vi "Autonomous Independent.vi"() -> ()   [LabVIEW 2011]
doc: "This VI is called when autonomous begins, and will automatically be terminated when autonomous ends. You can carry out timed or sensor driven robot movement independently without needing to return to the caller."
uses:
  Autonomous Mode Selector.ctl
  <vilib>/Rock Robotics/WPI/Solenoid/WPI_SolenoidValue.ctl
  Shared/Autonomous Recording TypeDef.ctl
  Robot Global Data.vi
  Shooter Global.vi
  <vilib>/Rock Robotics/WPI/Solenoid/WPI_SolenoidSetEnum.vi
  <vilib>/addons/control/pid/pid.llb/PID (DBL).vi
  <vilib>/addons/control/pid/NI_PID_pid.lvlib
panel:
  in  "PID gains":T1={"proportional gain (Kc)"=0.01, "integral time (Ti, min)"=0.1, "derivative time (Td, min)"=0.0}
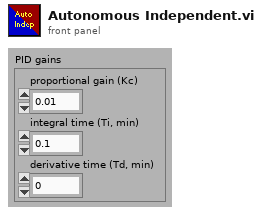
[diagram p1: front panel]
types:
  T1 = cluster{"proportional gain (Kc)":dbl, "integral time (Ti, min)":dbl, "derivative time (Td, min)":dbl}
  T2 = typedef "Autonomous Mode Selector.ctl" = enum16{"Shoot", "No Autonomous", "Shoot & Move"}
  T3 = typedef "WPI_DigitalInputDevRef.ctl" = cluster{"DevStatus":errorcluster, "DIO Channel":T4, "Digital Module":T5}
  T4 = typedef "FPGA_DIOChannel.ctl" = enum8{"DIO 1", "DIO 2", "DIO 3", "DIO 4", "DIO 5", "DIO 6", "DIO 7", "DIO 8", "DIO 9", "DIO 10", "DIO 11", "DIO 12", "DIO 13", "DIO 14", "Invalid"}
  T5 = typedef "FPGA_TypedefDigitalModule.ctl" = enum16{"Digital Module 1", "Digital Module 2"}
  T6 = enum16{"Off", "Open Loop Control", "Closed Loop Control", "Top Spin"}
  T7 = typedef "WPI_SolenoidValue.ctl" = enum16{"Off", "On", "Forward", "Reverse"}
  T8 = typedef "WPI_SolenoidDevRef.ctl" = cluster{"DevStatus":errorcluster, "Solenoid Module":T9, "Forward Solenoid Channel":T10, "Reverse Solenoid Channel":T10}
  T9 = typedef "FPGA_TypedefSolenoidModule.ctl" = enum16{"Solenoid Module 1", "Solenoid Module 2"}
  T10 = typedef "WPI_SolenoidChannel.ctl" = enum8{"Solenoid 1", "Solenoid 2", "Solenoid 3", "Solenoid 4", "Solenoid 5", "Solenoid 6", "Solenoid 7", "Solenoid 8", "Invalid"}
  T11 = typedef "WPI_RobotDriveDevRef.ctl" = cluster{"DevStatus":errorcluster, "Motors[]":T12[], "Square Inputs":bool, "Max Output":dbl, "Isochronous":bool}
  T12 = typedef "WPI_MotorControlDeviceRef.ctl" = cluster{"DeviceStatus":errorcluster, "Type":enum16{"PWM", "CAN"}, "PWM":cluster{"Digital Module":T5, "PWM Channel":T13, "DeadBand":T14}, "CAN":cluster{"Device Number":u8, "Control Mode":T15, "Semaphore":T16, "Max Vout":dbl}, "Invert":bool, "TransformRef":T17, "InvTransformRef":T17}
  T13 = typedef "FPGA_DIOPWMChannel.ctl" = enum8{"PWM 1", "PWM 2", "PWM 3", "PWM 4", "PWM 5", "PWM 6", "PWM 7", "PWM 8", "PWM 9", "PWM 10", "Invalid"}
  T14 = typedef "WPI_PWMDeadband.ctl" = cluster{"Name":string, "maxPositivePwm":i32, "minPositivePwm":i32, "centerPwm":i32, "maxNegativePwm":i32, "minNegativePwm":i32, "angularRange":u16}
  T15 = typedef "WPI_CANJaguar_ControlMode.ctl" = enum8{"Percent VBus", "Current", "Speed", "Position", "Voltage"}
  T16 = typedef "Semaphore RefNum" = refnum<k1>
  T17 = typedef "WPI_PWMTransform_ConPane.ctl" = refnum<vi>
  T18 = typedef "Autonomous Recording TypeDef.ctl" = cluster{"Left Drive Encoder":dbl, "Right Drive Encoder":dbl, "Shooter Mode":enum16{"Off", "Open Loop Control", "Closed Loop Control", "Top Spin"}, "Set RPM":dbl, "Set Motor Speed":dbl, "Horn":bool, "Shift Low":bool, "Shift High":bool, "Fire":bool, "Reset Encoders":bool}
  T19 = typedef "WPI_EncoderDevRef.ctl" = cluster{"DevStatus":errorcluster, "EncoderIndex":T20, "CounterIndex":T21, "DistancePerCount":dbl, "Decoding Type":T22}
  T20 = typedef "FPGA_EncoderIdx.ctl" = enum8{"Enc 0", "Enc 1", "Enc 2", "Enc 3", "Invalid"}
  T21 = typedef "FPGA_CounterCtrSystemIndex.ctl" = enum8{"Ctr 0", "Ctr 1", "Ctr 2", "Ctr 3", "Ctr 4", "Ctr 5", "Ctr 6", "Ctr 7", "Invalid"}
  T22 = typedef "WPI_EncoderType.ctl" = enum16{"1x", "2x", "4x"}
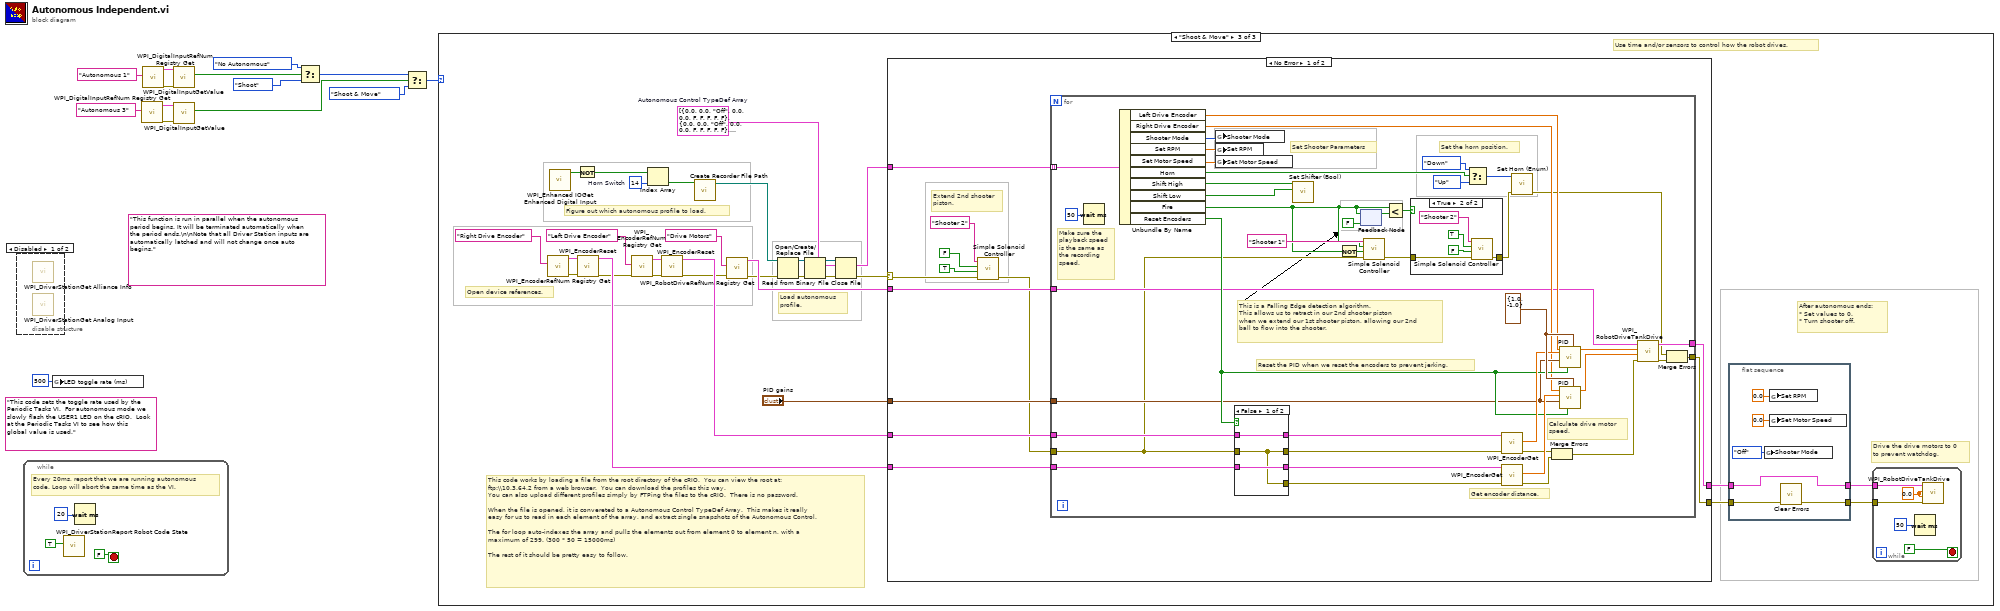
[diagram p0: block diagram]
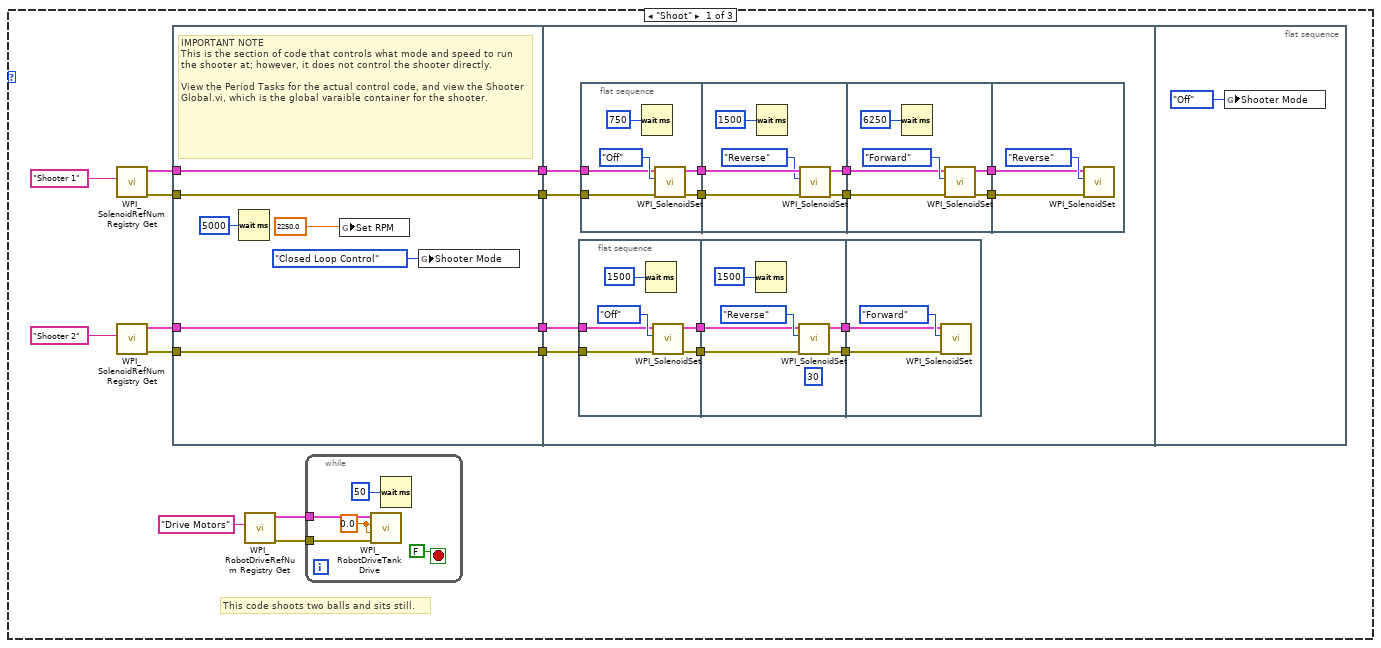
[diagram p3: hidden frame]
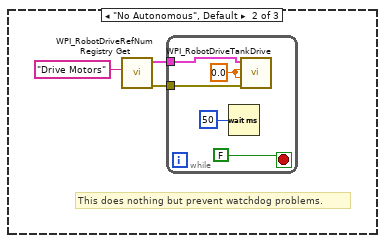
[diagram p4: hidden frame]
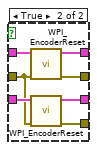
[diagram p6: hidden frame]
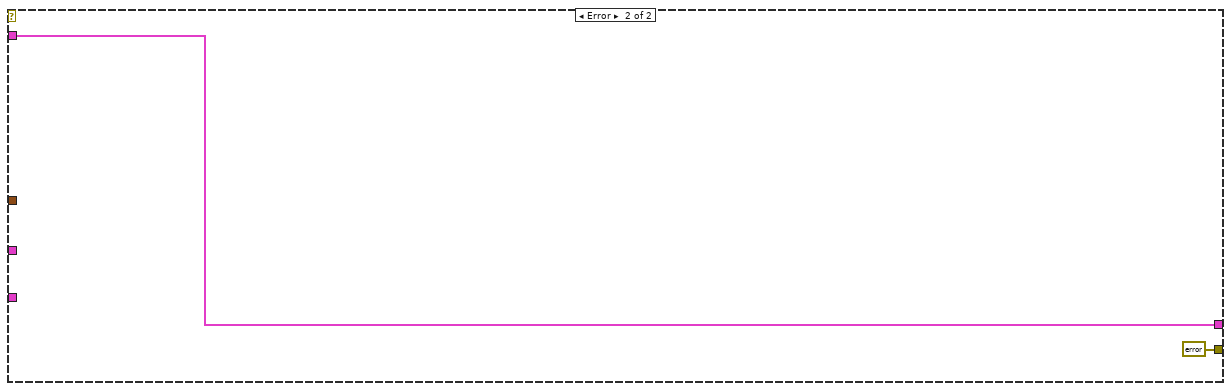
[diagram p7: hidden frame]
diagram:
  (unwired) "This code sets the toggle rate used by the Periodic Tasks VI.  For autonomous mode we slowly flash the USER1 LED on the cRIO.  Look at the Periodic Tasks VI to see how this global value is used."
  (unwired) "This function is run in parallel when the autonomous period begins. It will be terminated automatically when the period ends.\n\nNote that all Driver Station inputs are automatically latched and will not change once auto begins."
  # "Use time and/or sensors to control how the robot drives."
  n1 = disable-structure shown="Disabled" {
    frame Disabled {
      n2 = call <vilib>:"WPI_DriverStationGet Alliance Info.vi"() -> ()  [unwired: 12 out]
      n3 = call <vilib>:"WPI_DriverStationGet Analog Input.vi"() -> ()  [unwired: 12 out]
    }
    frame Enabled {
    }
  }
  n4 = while {
    stop <- FALSE stop-if-true
    # "Every 20ms, report that we are running autonomous\ncode. Loop will abort the same time as the VI."
    n5 = call <vilib>:"WPI_DriverStationReport Robot Code State.vi"("Autonomous"=TRUE) -> ()  [unwired: 10 in, 1 out]
    n6 = Wait (ms)(milliseconds to wait=u32 20) -> ()  [unwired: 1 out]
  }
  n7 = global write "Robot Global Data.vi" "LED toggle rate (ms)"(u32 500 ("LED ms toggle rate")) -> ()
  n8 = call <vilib>:"WPI_DigitalInputRefNum Registry Get.vi"("refnum name"="Autonomous 3") -> ("error out"=w9:errorcluster, "DigitalInputDevRef"=w8:T3)  [unwired: 9 in]
  n9 = call <vilib>:"WPI_DigitalInputRefNum Registry Get.vi"("refnum name"="Autonomous 1") -> ("error out"=w11:errorcluster, "DigitalInputDevRef"=w10:T3)  [unwired: 9 in]
  n10 = call <vilib>:"WPI_DigitalInputGetValue.vi"("error in (no error)"=w11, "DigitalInputDevRef"=w10) -> ("Value"=w7:bool)  [unwired: 7 in, 2 out]
  n11 = call <vilib>:"WPI_DigitalInputGetValue.vi"("error in (no error)"=w9, "DigitalInputDevRef"=w8) -> ("Value"=w2:bool)  [unwired: 7 in, 2 out]
  n12 = Select(t=Autonomous_Mode_Selector."No Autonomous", s=w7, f=Autonomous_Mode_Selector."Shoot") -> (s? t:f=w3:T2)
  n13 = Select(t=w3, s=w2, f=Autonomous_Mode_Selector."Shoot & Move") -> (s? t:f=w1:T2)
  n14 = case shown="\"Shoot & Move\"" w1 {
    frame "Shoot" {
      # "This code shoots two balls and sits still."
      n15 = call <vilib>:"WPI_SolenoidRefNum Registry Get.vi"("refnum name"="Shooter 1") -> ("error out"=w22:errorcluster, "SolenoidDevRef"=w24:T8)  [unwired: 9 in]
      n16 = call <vilib>:"WPI_SolenoidRefNum Registry Get.vi"("refnum name"="Shooter 2") -> ("error out"=w18:errorcluster, "SolenoidDevRef"=w20:T8)  [unwired: 9 in]
      n17 = flat-sequence {
        tunnel: [w34] -> w25
        tunnel: w24 -> [w34]
        tunnel: [w33] -> w23
        tunnel: w22 -> [w33]
        tunnel: [w32] -> w21
        tunnel: w20 -> [w32]
        tunnel: [w31] -> w19
        tunnel: w18 -> [w31]
        tunnel: w25 -> [w41]
        tunnel: w23 -> [w40]
        tunnel: w21 -> [w39]
        tunnel: w19 -> [w38]
        frame #0 {
          # "IMPORTANT NOTE\nThis is the section of code that controls what mode and speed to run the shooter at; however, it does not control the shooter directly.\n\nView the Period Tasks for the actual control code, and view the Shooter Global.vi, which is the global varaible container for the shooter."
          n18 = Wait (ms)(milliseconds to wait=u32 5000) -> ()  [unwired: 1 out]
          n19 = global write "Shooter Global.vi" "Set RPM"(2250.0 ("Output")) -> ()
          n20 = global write "Shooter Global.vi" "Shooter Mode"(T6."Closed Loop Control" ("Shooter Mode")) -> ()
        }
        frame #1 {
          n21 = flat-sequence {
            tunnel: w39 -> [w56]
            tunnel: w38 -> [w55]
            tunnel: [w53] -> w45
            tunnel: [w52] -> w44
            tunnel: w45 -> [w61]
            tunnel: w44 -> [w60]
            tunnel: [w59] -> w43
            tunnel: [w58] -> w42
            tunnel: w43 -> [w65]
            tunnel: w42 -> [w64]
            frame #0 {
              n22 = Wait (ms)(milliseconds to wait=u32 1500) -> ()  [unwired: 1 out]
              n23 = call-poly <vilib>:"WPI_SolenoidSet.vi"("error in (no error)"=w55, "Value"=WPI_SolenoidValue."Off", "SolenoidDevRef"=w56) -> ("error out"=w52:errorcluster, "SolenoidDevRef"=w53:T8)  [unwired: 7 in]
            }
            frame #1 {
              (unwired) 30 ("y")
              n24 = Wait (ms)(milliseconds to wait=u32 1500) -> ()  [unwired: 1 out]
              n25 = call-poly <vilib>:"WPI_SolenoidSet.vi"("error in (no error)"=w60, "Value"=WPI_SolenoidValue."Reverse", "SolenoidDevRef"=w61) -> ("error out"=w58:errorcluster, "SolenoidDevRef"=w59:T8)  [unwired: 7 in]
            }
            frame #2 {
              n26 = call-poly <vilib>:"WPI_SolenoidSet.vi"("error in (no error)"=w64, "Value"=WPI_SolenoidValue."Forward", "SolenoidDevRef"=w65) -> ()  [unwired: 7 in, 2 out]
            }
          }
          n27 = flat-sequence {
            tunnel: w41 -> [w71]
            tunnel: w40 -> [w70]
            tunnel: [w68] -> w51
            tunnel: [w67] -> w50
            tunnel: w51 -> [w78]
            tunnel: w50 -> [w77]
            tunnel: [w74] -> w49
            tunnel: [w73] -> w48
            tunnel: w49 -> [w83]
            tunnel: w48 -> [w82]
            tunnel: [w80] -> w47
            tunnel: [w79] -> w46
            tunnel: w47 -> [w86]
            tunnel: w46 -> [w85]
            frame #0 {
              n28 = Wait (ms)(milliseconds to wait=u32 750) -> ()  [unwired: 1 out]
              n29 = call-poly <vilib>:"WPI_SolenoidSet.vi"("error in (no error)"=w70, "Value"=WPI_SolenoidValue."Off", "SolenoidDevRef"=w71) -> ("error out"=w67:errorcluster, "SolenoidDevRef"=w68:T8)  [unwired: 7 in]
            }
            frame #1 {
              n30 = Wait (ms)(milliseconds to wait=u32 1500) -> ()  [unwired: 1 out]
              n31 = call-poly <vilib>:"WPI_SolenoidSet.vi"("error in (no error)"=w77, "Value"=WPI_SolenoidValue."Reverse", "SolenoidDevRef"=w78) -> ("error out"=w73:errorcluster, "SolenoidDevRef"=w74:T8)  [unwired: 7 in]
            }
            frame #2 {
              n32 = Wait (ms)(milliseconds to wait=u32 6250) -> ()  [unwired: 1 out]
              n33 = call-poly <vilib>:"WPI_SolenoidSet.vi"("error in (no error)"=w82, "Value"=WPI_SolenoidValue."Forward", "SolenoidDevRef"=w83) -> ("error out"=w79:errorcluster, "SolenoidDevRef"=w80:T8)  [unwired: 7 in]
            }
            frame #3 {
              n34 = call-poly <vilib>:"WPI_SolenoidSet.vi"("error in (no error)"=w85, "Value"=WPI_SolenoidValue."Reverse", "SolenoidDevRef"=w86) -> ()  [unwired: 7 in, 2 out]
            }
          }
        }
        frame #2 {
          n35 = global write "Shooter Global.vi" "Shooter Mode"(T6."Off" ("Shooter Mode")) -> ()
        }
      }
      n36 = call <vilib>:"WPI_RobotDriveRefNum Registry Get.vi"("refnum name"="Drive Motors") -> ("error out"=w29:errorcluster, "RobotDriveDevRef"=w28:T11)  [unwired: 9 in]
      n37 = while {
        tunnel: w29 -> [w91]
        tunnel: w28 -> [w90]
        stop <- FALSE stop-if-true
        w89 = 0.0 ("Left axis value")
        n38 = call <vilib>:"WPI_RobotDriveTankDrive.vi"("error in (no error)"=w91, "Right axis value"=w89, "Left axis value"=w89, "RobotDriveDevRef"=w90) -> ()  [unwired: 6 in, 2 out]
        n39 = Wait (ms)(milliseconds to wait=u32 50) -> ()  [unwired: 1 out]
      }
    }
    frame "No Autonomous", Default {
      # "This does nothing but prevent watchdog problems."
      n40 = call <vilib>:"WPI_RobotDriveRefNum Registry Get.vi"("refnum name"="Drive Motors") -> ("error out"=w94:errorcluster, "RobotDriveDevRef"=w95:T11)  [unwired: 9 in]
      n41 = while {
        tunnel: w95 -> [w101]
        tunnel: w94 -> [w97]
        stop <- FALSE stop-if-true
        w100 = 0.0 ("Left axis value")
        n42 = Wait (ms)(milliseconds to wait=u32 50) -> ()  [unwired: 1 out]
        n43 = call <vilib>:"WPI_RobotDriveTankDrive.vi"("error in (no error)"=w97, "Right axis value"=w100, "Left axis value"=w100, "RobotDriveDevRef"=w101) -> ()  [unwired: 6 in, 2 out]
      }
    }
    frame "Shoot & Move" {
      w108 = 14  # Horn Switch
      w115 = T18[] [{"Left Drive Encoder"=0.0, "Right Drive Encoder"=0.0, "Shooter Mode"=enum."Off", "Set RPM"=0.0, "Set Motor Speed"=0.0, "Horn"=FALSE, "Shift Low"=FALSE, "Shift High"=FALSE, "Fire"=FALSE, "Reset Encoders"=FALSE}, {"Left Drive Encoder"=0.0, "Right Drive Encoder"=0.0, "Shooter Mode"=enum."Off", "Set RPM"=0.0, "Set Motor Speed"=0.0, "Horn"=FALSE, "Shift Low"=FALSE, "Shift High"=FALSE, "Fire"=FALSE, "Reset Encoders"=FALSE}, {"Left Drive Encoder"=0.0, "Right Drive Encoder"=0.0, "Shooter Mode"=enum."Off", "Set RPM"=0.0, "Set Motor Speed"=0.0, "Horn"=FALSE, "Shift Low"=FALSE, "Shift High"=FALSE, "Fire"=FALSE, "Reset Encoders"=FALSE}, {"Left Drive Encoder"=0.0, "Right Drive Encoder"=0.0, "Shooter Mode"=enum."Off", "Set RPM"=0.0, "Set Motor Speed"=0.0, "Horn"=FALSE, "Shift Low"=FALSE, "Shift High"=FALSE, "Fire"=FALSE, "Reset Encoders"=FALSE}, {"Left Drive Encoder"=0.0, "Right Drive Encoder"=0.0, "Shooter Mode"=enum."Off", "Set RPM"=0.0, "Set Motor Speed"=0.0, "Horn"=FALSE, "Shift Low"=FALSE, "Shift High"=FALSE, "Fire"=FALSE, "Reset Encoders"=FALSE}, {"Left Drive Encoder"=0.0, "Right Drive Encoder"=0.0, "Shooter Mode"=enum."Off", "Set RPM"=0.0, "Set Motor Speed"=0.0, "Horn"=FALSE, "Shift Low"=FALSE, "Shift High"=FALSE, "Fire"=FALSE, "Reset Encoders"=FALSE}, {"Left Drive Encoder"=0.0, "Right Drive Encoder"=0.0, "Shooter Mode"=enum."Off", "Set RPM"=0.0, "Set Motor Speed"=0.0, "Horn"=FALSE, "Shift Low"=FALSE, "Shift High"=FALSE, "Fire"=FALSE, "Reset Encoders"=FALSE}, {"Left Drive Encoder"=0.0, "Right Drive Encoder"=0.0, "Shooter Mode"=enum."Off", "Set RPM"=0.0, "Set Motor Speed"=0.0, "Horn"=FALSE, "Shift Low"=FALSE, "Shift High"=FALSE, "Fire"=FALSE, "Reset Encoders"=FALSE}, {"Left Drive Encoder"=0.0, "Right Drive Encoder"=0.0, "Shooter Mode"=enum."Off", "Set RPM"=0.0, "Set Motor Speed"=0.0, "Horn"=FALSE, "Shift Low"=FALSE, "Shift High"=FALSE, "Fire"=FALSE, "Reset Encoders"=FALSE}, {"Left Drive Encoder"=0.0, "Right Drive Encoder"=0.0, "Shooter Mode"=enum."Off", "Set RPM"=0.0, "Set Motor Speed"=0.0, "Horn"=FALSE, "Shift Low"=FALSE, "Shift High"=FALSE, "Fire"=FALSE, "Reset Encoders"=FALSE}, {"Left Drive Encoder"=0.0, "Right Drive Encoder"=0.0, "Shooter Mode"=enum."Off", "Set RPM"=0.0, "Set Motor Speed"=0.0, "Horn"=FALSE, "Shift Low"=FALSE, "Shift High"=FALSE, "Fire"=FALSE, "Reset Encoders"=FALSE}, {"Left Drive Encoder"=0.0, "Right Drive Encoder"=0.0, "Shooter Mode"=enum."Off", "Set RPM"=0.0, "Set Motor Speed"=0.0, "Horn"=FALSE, "Shift Low"=FALSE, "Shift High"=FALSE, "Fire"=FALSE, "Reset Encoders"=FALSE}, {"Left Drive Encoder"=0.0, "Right Drive Encoder"=0.0, "Shooter Mode"=enum."Off", "Set RPM"=0.0, "Set Motor Speed"=0.0, "Horn"=FALSE, "Shift Low"=FALSE, "Shift High"=FALSE, "Fire"=FALSE, "Reset Encoders"=FALSE}, {"Left Drive Encoder"=0.0, "Right Drive Encoder"=0.0, "Shooter Mode"=enum."Off", "Set RPM"=0.0, "Set Motor Speed"=0.0, "Horn"=FALSE, "Shift Low"=FALSE, "Shift High"=FALSE, "Fire"=FALSE, "Reset Encoders"=FALSE}, {"Left Drive Encoder"=0.0, "Right Drive Encoder"=0.0, "Shooter Mode"=enum."Off", "Set RPM"=0.0, "Set Motor Speed"=0.0, "Horn"=FALSE, "Shift Low"=FALSE, "Shift High"=FALSE, "Fire"=FALSE, "Reset Encoders"=FALSE}, {"Left Drive Encoder"=0.0, "Right Drive Encoder"=0.0, "Shooter Mode"=enum."Off", "Set RPM"=0.0, "Set Motor Speed"=0.0, "Horn"=FALSE, "Shift Low"=FALSE, "Shift High"=FALSE, "Fire"=FALSE, "Reset Encoders"=FALSE}, {"Left Drive Encoder"=0.0, "Right Drive Encoder"=0.0, "Shooter Mode"=enum."Off", "Set RPM"=0.0, "Set Motor Speed"=0.0, "Horn"=FALSE, "Shift Low"=FALSE, "Shift High"=FALSE, "Fire"=FALSE, "Reset Encoders"=FALSE}, {"Left Drive Encoder"=0.0, "Right Drive Encoder"=0.0, "Shooter Mode"=enum."Off", "Set RPM"=0.0, "Set Motor Speed"=0.0, "Horn"=FALSE, "Shift Low"=FALSE, "Shift High"=FALSE, "Fire"=FALSE, "Reset Encoders"=FALSE}, {"Left Drive Encoder"=0.0, "Right Drive Encoder"=0.0, "Shooter Mode"=enum."Off", "Set RPM"=0.0, "Set Motor Speed"=0.0, "Horn"=FALSE, "Shift Low"=FALSE, "Shift High"=FALSE, "Fire"=FALSE, "Reset Encoders"=FALSE}, {"Left Drive Encoder"=0.0, "Right Drive Encoder"=0.0, "Shooter Mode"=enum."Off", "Set RPM"=0.0, "Set Motor Speed"=0.0, "Horn"=FALSE, "Shift Low"=FALSE, "Shift High"=FALSE, "Fire"=FALSE, "Reset Encoders"=FALSE}, {"Left Drive Encoder"=0.0, "Right Drive Encoder"=0.0, "Shooter Mode"=enum."Off", "Set RPM"=0.0, "Set Motor Speed"=0.0, "Horn"=FALSE, "Shift Low"=FALSE, "Shift High"=FALSE, "Fire"=FALSE, "Reset Encoders"=FALSE}, {"Left Drive Encoder"=0.0, "Right Drive Encoder"=0.0, "Shooter Mode"=enum."Off", "Set RPM"=0.0, "Set Motor Speed"=0.0, "Horn"=FALSE, "Shift Low"=FALSE, "Shift High"=FALSE, "Fire"=FALSE, "Reset Encoders"=FALSE}, {"Left Drive Encoder"=0.0, "Right Drive Encoder"=0.0, "Shooter Mode"=enum."Off", "Set RPM"=0.0, "Set Motor Speed"=0.0, "Horn"=FALSE, "Shift Low"=FALSE, "Shift High"=FALSE, "Fire"=FALSE, "Reset Encoders"=FALSE}, {"Left Drive Encoder"=0.0, "Right Drive Encoder"=0.0, "Shooter Mode"=enum."Off", "Set RPM"=0.0, "Set Motor Speed"=0.0, "Horn"=FALSE, "Shift Low"=FALSE, "Shift High"=FALSE, "Fire"=FALSE, "Reset Encoders"=FALSE}, {"Left Drive Encoder"=0.0, "Right Drive Encoder"=0.0, "Shooter Mode"=enum."Off", "Set RPM"=0.0, "Set Motor Speed"=0.0, "Horn"=FALSE, "Shift Low"=FALSE, "Shift High"=FALSE, "Fire"=FALSE, "Reset Encoders"=FALSE}, {"Left Drive Encoder"=0.0, "Right Drive Encoder"=0.0, "Shooter Mode"=enum."Off", "Set RPM"=0.0, "Set Motor Speed"=0.0, "Horn"=FALSE, "Shift Low"=FALSE, "Shift High"=FALSE, "Fire"=FALSE, "Reset Encoders"=FALSE}, {"Left Drive Encoder"=0.0, "Right Drive Encoder"=0.0, "Shooter Mode"=enum."Off", "Set RPM"=0.0, "Set Motor Speed"=0.0, "Horn"=FALSE, "Shift Low"=FALSE, "Shift High"=FALSE, "Fire"=FALSE, "Reset Encoders"=FALSE}, {"Left Drive Encoder"=0.0, "Right Drive Encoder"=0.0, "Shooter Mode"=enum."Off", "Set RPM"=0.0, "Set Motor Speed"=0.0, "Horn"=FALSE, "Shift Low"=FALSE, "Shift High"=FALSE, "Fire"=FALSE, "Reset Encoders"=FALSE}, {"Left Drive Encoder"=0.0, "Right Drive Encoder"=0.0, "Shooter Mode"=enum."Off", "Set RPM"=0.0, "Set Motor Speed"=0.0, "Horn"=FALSE, "Shift Low"=FALSE, "Shift High"=FALSE, "Fire"=FALSE, "Reset Encoders"=FALSE}, {"Left Drive Encoder"=0.0, "Right Drive Encoder"=0.0, "Shooter Mode"=enum."Off", "Set RPM"=0.0, "Set Motor Speed"=0.0, "Horn"=FALSE, "Shift Low"=FALSE, "Shift High"=FALSE, "Fire"=FALSE, "Reset Encoders"=FALSE}, {"Left Drive Encoder"=0.0, "Right Drive Encoder"=0.0, "Shooter Mode"=enum."Off", "Set RPM"=0.0, "Set Motor Speed"=0.0, "Horn"=FALSE, "Shift Low"=FALSE, "Shift High"=FALSE, "Fire"=FALSE, "Reset Encoders"=FALSE}, {"Left Drive Encoder"=0.0, "Right Drive Encoder"=0.0, "Shooter Mode"=enum."Off", "Set RPM"=0.0, "Set Motor Speed"=0.0, "Horn"=FALSE, "Shift Low"=FALSE, "Shift High"=FALSE, "Fire"=FALSE, "Reset Encoders"=FALSE}, {"Left Drive Encoder"=0.0, "Right Drive Encoder"=0.0, "Shooter Mode"=enum."Off", "Set RPM"=0.0, "Set Motor Speed"=0.0, "Horn"=FALSE, "Shift Low"=FALSE, "Shift High"=FALSE, "Fire"=FALSE, "Reset Encoders"=FALSE}, {"Left Drive Encoder"=0.0, "Right Drive Encoder"=0.0, "Shooter Mode"=enum."Off", "Set RPM"=0.0, "Set Motor Speed"=0.0, "Horn"=FALSE, "Shift Low"=FALSE, "Shift High"=FALSE, "Fire"=FALSE, "Reset Encoders"=FALSE}, {"Left Drive Encoder"=0.0, "Right Drive Encoder"=0.0, "Shooter Mode"=enum."Off", "Set RPM"=0.0, "Set Motor Speed"=0.0, "Horn"=FALSE, "Shift Low"=FALSE, "Shift High"=FALSE, "Fire"=FALSE, "Reset Encoders"=FALSE}, {"Left Drive Encoder"=-1.7999999999999998, "Right Drive Encoder"=-1.7999999999999998, "Shooter Mode"=enum."Off", "Set RPM"=0.0, "Set Motor Speed"=0.0, "Horn"=FALSE, "Shift Low"=FALSE, "Shift High"=FALSE, "Fire"=FALSE, "Reset Encoders"=FALSE}, {"Left Drive Encoder"=-8.64, "Right Drive Encoder"=-6.12, "Shooter Mode"=enum."Off", "Set RPM"=0.0, "Set Motor Speed"=0.0, "Horn"=FALSE, "Shift Low"=FALSE, "Shift High"=FALSE, "Fire"=FALSE, "Reset Encoders"=FALSE}, {"Left Drive Encoder"=-14.399999999999999, "Right Drive Encoder"=-13.68, "Shooter Mode"=enum."Off", "Set RPM"=0.0, "Set Motor Speed"=0.0, "Horn"=FALSE, "Shift Low"=FALSE, "Shift High"=FALSE, "Fire"=FALSE, "Reset Encoders"=FALSE}, {"Left Drive Encoder"=-24.119999999999997, "Right Drive Encoder"=-27.36, "Shooter Mode"=enum."Off", "Set RPM"=0.0, "Set Motor Speed"=0.0, "Horn"=FALSE, "Shift Low"=FALSE, "Shift High"=FALSE, "Fire"=FALSE, "Reset Encoders"=FALSE}, {"Left Drive Encoder"=-36.36, "Right Drive Encoder"=0.0, "Shooter Mode"=enum."Off", "Set RPM"=0.0, "Set Motor Speed"=0.0, "Horn"=FALSE, "Shift Low"=FALSE, "Shift High"=FALSE, "Fire"=FALSE, "Reset Encoders"=FALSE}]  # Autonomous Control TypeDef Array
      # "After autonomous ends:\n* Set values to 0.\n* Turn shooter off."
      # "This code works by loading a file from the root directory of the cRIO.  You can view the root at:\nftp:\\\\10.3.64.2 from a web browser.  You can download the profiles this way.\nYou can also upload different profiles simply by FTPing the files to the cRIO.  There is no password.\n\nWhen the file is opened, it is convereted to a Autonomous Control TypeDef Array.  This makes it really\neasy for us to read in each element of the array, and extract single snapshots of the Autonomous Control.\n\nThe for loop auto-indexes the array and pulls the elements out from element 0 to element n, with a \nmaximum of 299. (300 * 50 = 15000ms)\n\nThe rest of it should be pretty easy to follow."
      # "Drive the drive motors to 0\nto prevent watchdog."
      # "Figure out which autonomous profile to load."
      # "Load autonomous\nprofile."
      # "Open device references."
      n44 = call <vilib>:"WPI_EncoderRefNum Registry Get.vi"("refnum name"="Right Drive Encoder") -> ("error out"=w129:errorcluster, "EncoderDevRef"=w126:T19)  [unwired: 9 in]
      n45 = call <vilib>:"WPI_Enhanced IOGet Enhanced Digital Input.vi"() -> ("Digital Input [1-16]"=w106:bool[])  [unwired: 10 in, 1 out]
      n46 = Not(x=w106) -> (.not. x?=w107:bool[])
      n47 = call <vilib>:"WPI_EncoderReset.vi"("error in (no error)"=w129, "EncoderDevRef"=w126) -> ("error out"=w110:errorcluster, "EncoderDevRef"=w124:T19)  [unwired: 8 out]
      n48 = call <vilib>:"WPI_EncoderRefNum Registry Get.vi"("error in (no error)"=w110, "refnum name"="Left Drive Encoder") -> ("error out"=w128:errorcluster, "EncoderDevRef"=w127:T19)  [unwired: 8 in]
      n49 = Index Array(array=w107, index=w108) -> (element=w109:bool)
      n50 = call <vilib>:"WPI_EncoderReset.vi"("error in (no error)"=w128, "EncoderDevRef"=w127) -> ("error out"=w111:errorcluster, "EncoderDevRef"=w125:T19)  [unwired: 8 out]
      n51 = call "Create Recorder File Path.vi"("T: Move_Shoot\nF: Shoot_Move"=w109) -> ("Path"=w105:path)  [unwired: 10 in]
      n52 = call <vilib>:"WPI_RobotDriveRefNum Registry Get.vi"("error in (no error)"=w111, "refnum name"="Drive Motors") -> ("error out"=w121:errorcluster, "RobotDriveDevRef"=w122:T11)  [unwired: 8 in]
      n53 = Open/Create/Replace File(file path (use dialog)=w105, error in=w121) -> (refnum out=w116:refnum<file>, error out=w117:errorcluster)  [unwired: 4 in, 1 out]
      n54 = Read from Binary File(5:w115, 8:w117, 11:w116) -> (0:w112:errorcluster, 2:w114:T18[], 3:w113:refnum<file>)  [unwired: 3 in, 1 out]
      n55 = Close File(refnum=w113, error in=w112) -> (error out=w104:errorcluster)  [unwired: 1 out]
      n56 = case shown="No Error" w104 {
        selector: w104 -> [w134 _]
        tunnel: w125 -> [w143 _]
        tunnel: w124 -> [w142 _]
        tunnel: "PID gains" -> [w141 _]
        tunnel: w122 -> [w140 w204]
        tunnel: [w139 w204] -> w118
        tunnel: w114 -> [w138 _]
        tunnel: [w132 errorcluster {"status"=FALSE, "code"=0, "source"=""} ("error IO")] -> w102
        frame No Error {
          # "Extend 2nd shooter\npiston."
          n57 = call "Simple Solenoid Controller.vi"("error in (no error)"=w134, "Reverse"=TRUE, "Forward"=FALSE, "refnum name"="Shooter 2") -> ("error out"=w133:errorcluster)  [unwired: 6 in, 1 out]
          n58 = for {
            tunnel: w138 -> [w154] mode=indexing
            tunnel: w143 -> [w180]
            tunnel: w142 -> [w179]
            tunnel: w141 -> [w175]
            tunnel: w140 -> [w172]
            tunnel: [w155] -> w139
            tunnel: w133 -> [w151]
            tunnel: [w144] -> w132
            w185 = cluster{"output high":dbl, "output low":dbl} {"output high"=1.0, "output low"=-1.0} ("output range")
            # "Calculate drive motor\nspeed."
            # "Get encoder distance."
            # "Set the horn position."
            # "This is a Falling Edge detection algorithm.\nThis allows us to retract in our 2nd shooter piston\nwhen we extend our 1st shooter piston, allowing our 2nd\nball to flow into the shooter."
            # "Reset the PID when we reset the encoders to prevent jerking."
            # "Set Shooter Parameters"
            # "Make sure the\nplayback speed\nis the same as\nthe recording\nspeed."
            n59 = Wait (ms)(milliseconds to wait=u32 50) -> ()  [unwired: 1 out]
            n60 = Unbundle By Name(w154) -> ("Left Drive Encoder"=w174:dbl, "Right Drive Encoder"=w173:dbl, "Shooter Mode"=w156:T6, "Set RPM"=w158:dbl, "Set Motor Speed"=w157:dbl, "Horn"=w159:bool, "Shift High"=w171:bool, "Shift Low"=w170:bool, "Fire"=w165:bool, "Reset Encoders"=w176:bool)
            n61 = global write "Shooter Global.vi" "Shooter Mode"(w156) -> ()
            n62 = global write "Shooter Global.vi" "Set RPM"(w158) -> ()
            n63 = global write "Shooter Global.vi" "Set Motor Speed"(w157) -> ()
            n64 = case shown="False" w176 {
              tunnel: w180 -> [w195 w202]
              tunnel: w179 -> [w194 w201]
              tunnel: [w194 w200] -> w178
              tunnel: [w195 w199] -> w177
              tunnel: w151 -> [w193 w198]
              tunnel: [w193 w197] -> w153
              tunnel: [w193 w196] -> w152
              frame False {
              }
              frame True {
                n65 = call <vilib>:"WPI_EncoderReset.vi"("error in (no error)"=w198, "EncoderDevRef"=w202) -> ("error out"=w197:errorcluster, "EncoderDevRef"=w199:T19)  [unwired: 8 out]
                n66 = call <vilib>:"WPI_EncoderReset.vi"("error in (no error)"=w198, "EncoderDevRef"=w201) -> ("error out"=w196:errorcluster, "EncoderDevRef"=w200:T19)  [unwired: 8 out]
              }
            }
            n67 = call "Set Shifter (Bool).vi"("Low"=w170, "High"=w171) -> ()  [unwired: 9 in, 1 out]
            n68 = Not(x=w165) -> (.not. x?=w168:bool)
            n69 = feedback-in #1(w165) -> ()
            n70 = feedback #1(FALSE) -> (w164:bool)
            n71 = call "Simple Solenoid Controller.vi"("error in (no error)"=w151, "Reverse"=w168, "Forward"=w165, "refnum name"="Shooter 1") -> ("error out"=w167:errorcluster)  [unwired: 6 in, 1 out]
            n72 = Less?(x=w165, y=w164) -> (x < y?=w163:bool)
            n73 = case shown="True" w163 {
              tunnel: w167 -> [w187 w189]
              tunnel: [w187 w188] -> w146
              frame False {
              }
              frame True {
                n74 = call "Simple Solenoid Controller.vi"("error in (no error)"=w189, "Reverse"=FALSE, "Forward"=TRUE, "refnum name"="Shooter 2") -> ("error out"=w188:errorcluster)  [unwired: 6 in, 1 out]
              }
            }
            n75 = Select(t=enum16{"Down", "Up"}."Down" ("Horn"), s=w159, f=enum16{"Down", "Up"}."Up") -> (s? t:f=w162:enum16{"Down", "Up"})
            n76 = call <vilib>:"WPI_EncoderGet.vi"("error in (no error)"=w153, "EncoderDevRef"=w177) -> ("error out"=w150:errorcluster, "Distance"=w181:dbl)  [unwired: 8 out]
            n77 = call <vilib>:"WPI_EncoderGet.vi"("error in (no error)"=w152, "EncoderDevRef"=w178) -> ("error out"=w149:errorcluster, "Distance"=w182:dbl)  [unwired: 8 out]
            n78 = call "Set Horn (Enum).vi"("error in (no error)"=w146, "Horn"=w162) -> ("error out"=w145:errorcluster)  [unwired: 9 in]
            n79 = Merge Errors(w150, w149) -> (w148:errorcluster)
            n80 = call-poly <vilib>:"PID.vi"("reinitialize? (F)"=w176, "output range"=w185, "PID gains"=w175, "process variable"=w181, "setpoint"=w174) -> ("output"=w184:dbl)  [unwired: 5 in, 1 out]
            n81 = call-poly <vilib>:"PID.vi"("reinitialize? (F)"=w176, "output range"=w185, "PID gains"=w175, "process variable"=w182, "setpoint"=w173) -> ("output"=w183:dbl)  [unwired: 5 in, 1 out]
            n82 = call <vilib>:"WPI_RobotDriveTankDrive.vi"("error in (no error)"=w148, "Right axis value"=w183, "Left axis value"=w184, "RobotDriveDevRef"=w172) -> ("error out"=w147:errorcluster, "RobotDriveDevRef"=w155:T11)  [unwired: 6 in]
            n83 = Merge Errors(w145, w147) -> (w144:errorcluster)
          }
        }
        frame Error {
        }
      }
      n84 = flat-sequence {
        tunnel: [w208] -> w119
        tunnel: w118 -> [w208]
        tunnel: [w205] -> w103
        tunnel: w102 -> [w206]
        frame #0 {
          n85 = global write "Shooter Global.vi" "Shooter Mode"(T6."Off" ("Shooter Mode")) -> ()
          n86 = global write "Shooter Global.vi" "Set RPM"(0.0 ("Set RPM")) -> ()
          n87 = global write "Shooter Global.vi" "Set Motor Speed"(0.0 ("Set Motor Speed")) -> ()
          n88 = call <vilib>:"Clear Errors.vi"("error in (no error)"=w206) -> ("error out"=w205:errorcluster)  [unwired: 6 in]
        }
      }
      n89 = while {
        tunnel: w119 -> [w215]
        tunnel: w103 -> [w211]
        stop <- FALSE stop-if-true
        w214 = 0.0 ("Left axis value")
        n90 = Wait (ms)(milliseconds to wait=u32 50) -> ()  [unwired: 1 out]
        n91 = call <vilib>:"WPI_RobotDriveTankDrive.vi"("error in (no error)"=w211, "Right axis value"=w214, "Left axis value"=w214, "RobotDriveDevRef"=w215) -> ()  [unwired: 6 in, 2 out]
      }
    }
  }
